vi "WristControl.vi"(4 "Pivot Angle":dbl, 5 "Disable Wrist Forward":bool, 6 "Wrist Angle (relative to ground)":dbl, 7 "Disable Wrist Back":bool, 8 "error in (no error)":errorcluster, 9 "Wrist Multiplier (degrees/second)":dbl=0.07, 10 "Wrist Stick":cluster{"X":dbl, "Y":dbl}, 11 "MotorControlDevRef":T1={"DeviceStatus"={"status"=FALSE, "code"=0, "source"=""}, "Type"=enum."PWM", "PWM"={"Controller"=enum."Controller 1", "PWM Channel"=enum."Invalid", "DeadBand"={"Name"="", "maxPositivePwm"=0, "minPositivePwm"=0, "centerPwm"=0, "maxNegativePwm"=0, "minNegativePwm"=0, "angularRange"=0}}, "CAN"={"Device Number"=0, "Control Mode"=enum."Percent VBus", "Semaphore"=refnum, "Max Vout"=12.0, "TalonSRX Control Mode"=enum."Percent VBus"}, "Invert"=FALSE, "TransformRef"=refnum, "InvTransformRef"=refnum}) -> (0 "error out":errorcluster, 2 "Target Wrist Angle (relative to ground)":dbl, 3 "MotorControlDevRef":T1={"DeviceStatus"={"status"=FALSE, "code"=0, "source"=""}, "Type"=enum."PWM", "PWM"={"Controller"=enum."Controller 1", "PWM Channel"=enum."Invalid", "DeadBand"={"Name"="", "maxPositivePwm"=0, "minPositivePwm"=0, "centerPwm"=0, "maxNegativePwm"=0, "minNegativePwm"=0, "angularRange"=0}}, "CAN"={"Device Number"=0, "Control Mode"=enum."Percent VBus", "Semaphore"=refnum, "Max Vout"=12.0, "TalonSRX Control Mode"=enum."Percent VBus"}, "Invert"=FALSE, "TransformRef"=refnum, "InvTransformRef"=refnum})   [LabVIEW 2014]
uses:
  <vilib>/Rock Robotics/WPI/MotorControl/WPI_MotorControlDeviceRef.ctl
  <vilib>/Rock Robotics/WPI/MotorControl/WPI_MotorControlType.ctl
  <vilib>/Rock Robotics/SystemInterfaces/Typedef/FPGA_TypedefDigitalModule.ctl
  <vilib>/Rock Robotics/SystemInterfaces/DIO/FPGA_DIOPWMChannel.ctl
  <vilib>/Rock Robotics/WPI/PWM/WPI_PWMDeadband.ctl
  <vilib>/Rock Robotics/WPI/CAN/Jaguar/SubVIs/WPI_CANJaguar_ControlMode.ctl
  <vilib>/Rock Robotics/WPI/CAN/TalonSRX/WPI_CANTalonSRX_APIControlMode.ctl
  <vilib>/Rock Robotics/WPI/PWM/WPI_PWMTransform_ConPane.ctl
  Robot Global Data.vi
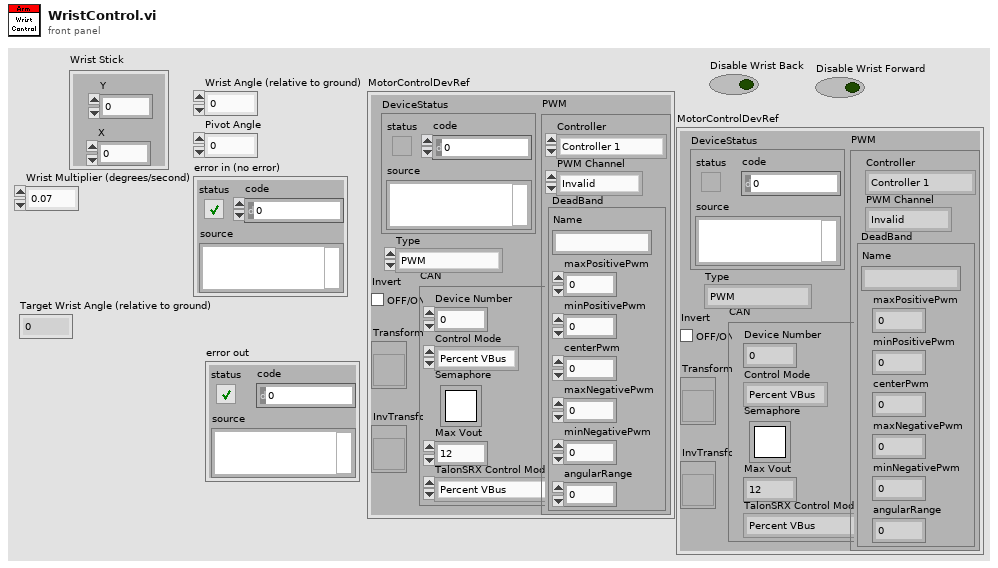
[diagram p1: front panel]
types:
  T1 = typedef "WPI_MotorControlDeviceRef.ctl" = cluster{"DeviceStatus":errorcluster, "Type":T2, "PWM":cluster{"Controller":T3, "PWM Channel":T4, "DeadBand":T5}, "CAN":cluster{"Device Number":u8, "Control Mode":T6, "Semaphore":T7, "Max Vout":dbl, "TalonSRX Control Mode":T8}, "Invert":bool, "TransformRef":T9, "InvTransformRef":T9}
  T2 = typedef "WPI_MotorControlType.ctl" = enum16{"PWM", "CAN", "CANTalonSRX"}
  T3 = typedef "FPGA_TypedefDigitalModule.ctl" = enum16{"Controller 1"}
  T4 = typedef "FPGA_DIOPWMChannel.ctl" = enum8{"PWM 0", "PWM 1", "PWM 2", "PWM 3", "PWM 4", "PWM 5", "PWM 6", "PWM 7", "PWM 8", "PWM 9", "PWM MXP 0", "PWM MXP 1", "PWM MXP 2", "PWM MXP 3", "PWM MXP 4", "PWM MXP 5", "PWM MXP 6", "PWM MXP 7", "PWM MXP 8", "PWM MXP 9", "Invalid"}
  T5 = typedef "WPI_PWMDeadband.ctl" = cluster{"Name":string, "maxPositivePwm":i32, "minPositivePwm":i32, "centerPwm":i32, "maxNegativePwm":i32, "minNegativePwm":i32, "angularRange":u16}
  T6 = typedef "WPI_CANJaguar_ControlMode.ctl" = enum8{"Percent VBus", "Current", "Speed", "Position", "Voltage"}
  T7 = typedef "Semaphore RefNum" = refnum<k1>
  T8 = typedef "WPI_CANTalonSRX_APIControlMode.ctl" = enum8{"Percent VBus", "Speed", "Position", "Slave", "Unchanged / Invalid"}
  T9 = typedef "WPI_PWMTransform_ConPane.ctl" = refnum<vi>
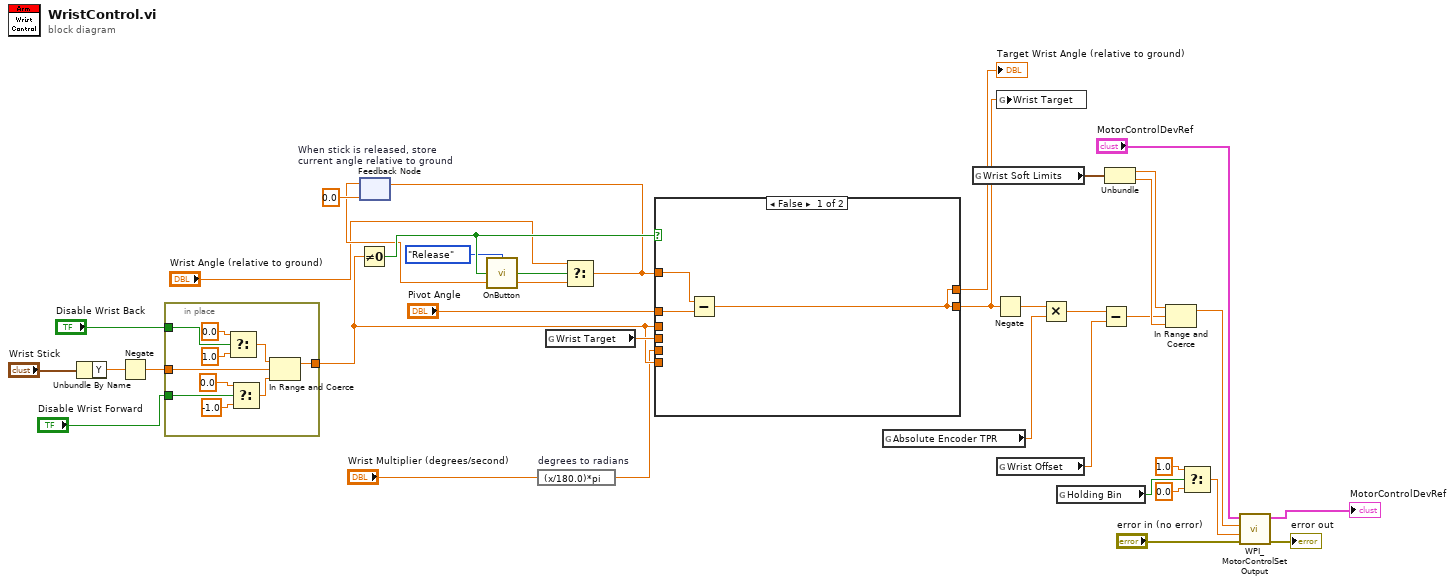
[diagram p0: block diagram]
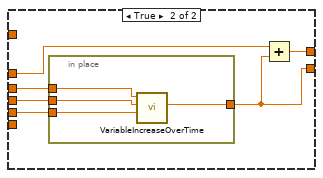
[diagram p2: hidden frame]
diagram:
  n1 = Unbundle By Name("Wrist Stick") -> ("Y"=w36:dbl)
  n2 = Negate(x=w36) -> (-x=w25:dbl)
  n3 = in-place {
    in-place-border: [w44] -> w2
    in-place-border: w25 -> [w43]
    in-place-border: "Disable Wrist Forward" -> [w38]
    in-place-border: "Disable Wrist Back" -> [w37]
    n4 = Select(t=0.0, s=w37, f=1.0) -> (s? t:f=w46:dbl)
    n5 = Select(t=0.0, s=w38, f=-1.0) -> (s? t:f=w45:dbl)
    n6 = In Range and Coerce(upper limit=w46, x=w43, lower limit=w45) -> (coerced(x)=w44:dbl)  [unwired: 1 out]
  }
  n7 = Not Equal To 0?(x=w2) -> (x != 0?=w33:bool)
  n8 = feedback #1 "When stick is released, store \ncurrent angle relative to ground"(0.0) -> (w23:dbl)
  n9 = call "OnButton.vi"("Button"=w33, "Mode"=enum16{"Press", "Release", "Both"}."Release") -> ("Value"=w24:bool)
  n10 = expression code="(x/180.0)*pi" "degrees to radians"("Wrist Multiplier (degrees/second)") -> (w1:dbl)
  n11 = global read "Robot Global Data.vi" "Wrist Target"() -> (w5:dbl)
  n12 = Select(t="Wrist Angle (relative to ground)", s=w24, f=w23) -> (s? t:f=w22:dbl)
  n13 = feedback-in #1(w22) -> ()
  n14 = case shown="False" w33 {
    tunnel: [w47 w51] -> w12
    tunnel: w22 -> [w49 _]
    tunnel: w2 -> [_ _]
    tunnel: "Pivot Angle" -> [w48 w52]
    tunnel: [w47 w50] -> w4
    tunnel: w5 -> [_ w54]
    tunnel: w2 -> [_ w55]
    tunnel: w1 -> [_ w53]
    frame False {
      n15 = Subtract(x=w49, y=w48) -> (x-y=w47:dbl)
    }
    frame True {
      n16 = in-place {
        in-place-border: w55 -> [w58]
        in-place-border: [w59] -> w50
        in-place-border: w54 -> [w57]
        in-place-border: w53 -> [w56]
        n17 = call "VariableIncreaseOverTime.vi"("Multiplier (units/sec)"=w56, "Variable in"=w57, "Joystick input"=w58) -> ("Variable out"=w59:dbl)  [unwired: 8 in]
      }
      n18 = Add(x=w52, y=w50) -> (x+y=w51:dbl)
    }
  }
  "Target Wrist Angle (relative to ground)" <- w12
  n19 = global read "Robot Global Data.vi" "Absolute Encoder TPR"() -> (w17:dbl)
  n20 = global read "Robot Global Data.vi" "Wrist Soft Limits"() -> (w21:cluster{"Forward":dbl, "Reverse":dbl})
  n21 = Negate(x=w4) -> (-x=w7:dbl)
  n22 = global write "Robot Global Data.vi" "Wrist Target"(w4) -> ()
  n23 = global read "Robot Global Data.vi" "Wrist Offset"() -> (w15:dbl)
  n24 = Multiply(x=w7, y=w17) -> (x*y=w16:dbl)
  n25 = global read "Robot Global Data.vi" "Holding Bin"() -> (w11:bool)
  n26 = Subtract(x=w16, y=w15) -> (x-y=w14:dbl)
  n27 = Unbundle(w21) -> ("Forward"=w19:dbl, "Reverse"=w20:dbl)
  n28 = In Range and Coerce(upper limit=w19, x=w14, lower limit=w20) -> (coerced(x)=w18:dbl)  [unwired: 1 out]
  n29 = Select(t=1.0, s=w11, f=0.0) -> (s? t:f=w8:dbl)
  n30 = call <vilib>:"WPI_MotorControlSetOutput.vi"("error in (no error)"="error in (no error)", "Sync Group / Parameter Slot"=w8, "Output"=w18, "MotorControlDevRef"="MotorControlDevRef") -> ("error out"=→"error out":errorcluster, "MotorControlDevRef"=→"MotorControlDevRef":T1)  [unwired: 5 in, 1 out]
